vi "TPNT_ChkError.vi"(8 "error in (no error)":errorcluster, 10 "testpoint In":T1={"name"="", "type"="", "algor"=[], "update_rate"=0.0, "Limits"={"Alarm Type"="", "Lower "=0.0, "Upper"=0.0, "Nominal"=0.0, "outrange"=FALSE, "Check"=TRUE, "latch"=FALSE, "level"=""}, "Samples"={"samples"=0, "counter"=0, "Values"=[], "Current Value"="", "filter"="", "precision"=2}, "next_update"=0, "Status"="", "monitor"=TRUE, "error"=FALSE, "Log"={"log"=FALSE, "file"=path "", "type"="", "format"="", "updaterate"=0.0, "nex_update"=0, "mode"=""}, "permissions"="", "ID"=""} {"Log"."updaterate" format="%.2f"; "Samples"."Values" format="%.2f"; "Samples"."samples" min=1 step=1; "Limits"."Nominal" format="%.2f"; "Limits"."Upper" format="%.2f"; "Limits"."Lower" format="%.2f"; "update_rate" format="%.2f"}) -> (0 "error out":errorcluster, 1 "error":bool, 2 "testpoint out":T1={"name"="", "type"="", "algor"=[], "update_rate"=0.0, "Limits"={"Alarm Type"="", "Lower "=0.0, "Upper"=0.0, "Nominal"=0.0, "outrange"=FALSE, "Check"=TRUE, "latch"=FALSE, "level"=""}, "Samples"={"samples"=0, "counter"=0, "Values"=[], "Current Value"="", "filter"="", "precision"=2}, "next_update"=0, "Status"="", "monitor"=TRUE, "error"=FALSE, "Log"={"log"=FALSE, "file"=path "", "type"="", "format"="", "updaterate"=0.0, "nex_update"=0, "mode"=""}, "permissions"="", "ID"=""} {"Log"."updaterate" format="%.2f"; "Samples"."Values" format="%.2f"; "Samples"."samples" min=1 step=1; "Limits"."Nominal" format="%.2f"; "Limits"."Upper" format="%.2f"; "Limits"."Lower" format="%.2f"; "update_rate" format="%.2f"})   [LabVIEW 2016]
uses:
  TPNT_TP.ctl
  TPNT_Limits.ctl
  TPNT_Samples.ctl
  TPNT_Log.ctl
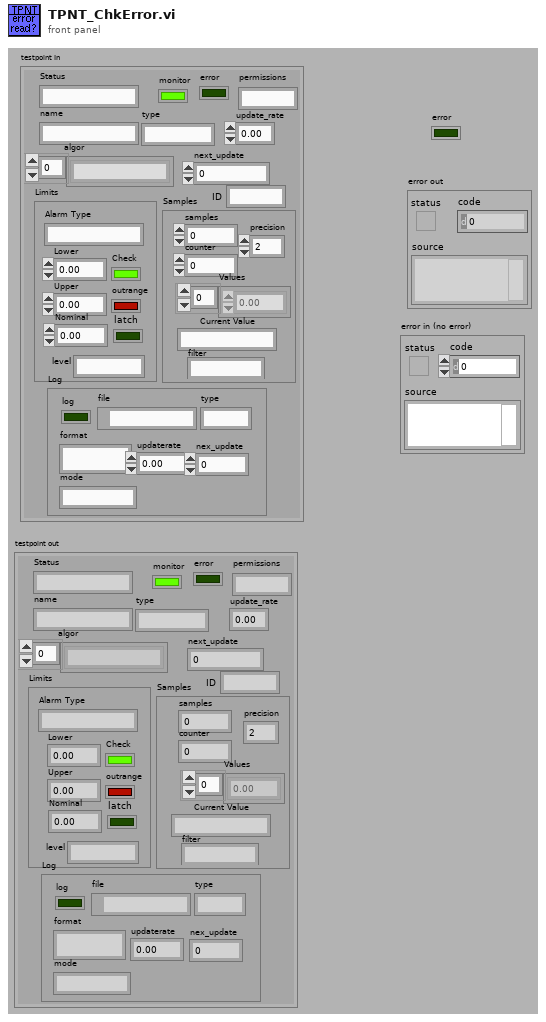
[diagram p1: front panel]
types:
  T1 = typedef "TPNT_TP.ctl" = cluster{"name":string, "type":string, "algor":string[], "update_rate":sgl, "Limits":T2, "Samples":T3, "next_update":u32, "Status":string, "monitor":bool, "error":bool, "Log":T4, "permissions":string, "ID":string}
  T2 = typedef "TPNT_Limits.ctl" = cluster{"Alarm Type":string, "Lower ":dbl, "Upper":dbl, "Nominal":dbl, "outrange":bool, "Check":bool, "latch":bool, "level":string}
  T3 = typedef "TPNT_Samples.ctl" = cluster{"samples":i32, "counter":i32, "Values":dbl[], "Current Value":string, "filter":string, "precision":u8}
  T4 = typedef "TPNT_Log.ctl" = cluster{"log":bool, "file":path, "type":string, "format":string, "updaterate":dbl, "nex_update":u32, "mode":string}
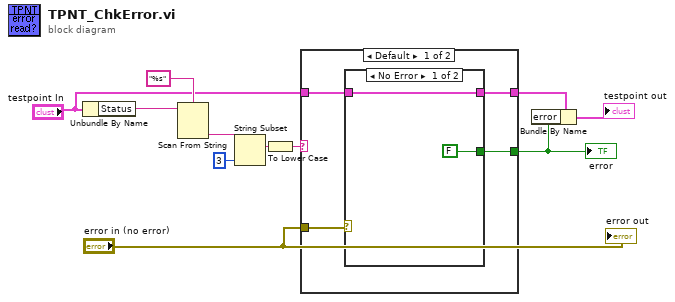
[diagram p0: block diagram]
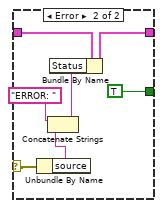
[diagram p2: hidden frame]
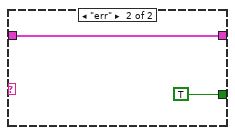
[diagram p3: hidden frame]
diagram:
  n1 = Unbundle By Name("testpoint In") -> ("Status"=w11:string)
  n2 = Scan From String(format string="%s", input string=w11) -> (output 1=w9:string)  [unwired: 2 in, 4 out]
  n3 = String Subset(string=w9, length (rest)=3 ("length (rest)")) -> (substring=w7:string)  [unwired: 1 out]
  n4 = To Lower Case(string=w7) -> (all lower case string=w6:string)
  n5 = case shown="Default" w6 {
    tunnel: "error in (no error)" -> [w15 _]
    tunnel: [w12 TRUE] -> w3
    tunnel: "testpoint In" -> [w14 w25]
    tunnel: [w13 w25] -> w2
    frame Default {
      n6 = case shown="No Error" w15 {
        selector: w15 -> [_ w22]
        tunnel: w14 -> [w16 w24]
        tunnel: [w16 w23] -> w13
        tunnel: [FALSE TRUE] -> w12
        frame No Error {
        }
        frame Error {
          n7 = Unbundle By Name(w22) -> ("source"=w20:string)
          n8 = Concatenate Strings("ERROR: " ("string"), w20) -> (w19:string)
          n9 = Bundle By Name(cluster=w24, "Status"=w19) -> (w23:T1)
        }
      }
    }
    frame "err" {
    }
  }
  "error" <- w3
  n10 = Bundle By Name(cluster=w2, "error"=w3) -> (→"testpoint out":T1)
  "error out" <- "error in (no error)"
